vi "DO redefine.vi"(6 "conninfo":T3={"host"="localhost", "port"="5432", "client_encoding"="WIN1251", "dbname"="data", "user"="postgres", "password"=""}, 7 "KFM":string[](array[string]), 8 "error in (no error)":errorcluster, 9 "DOParamTable":string="fdo_3", 10 "DOParameters":string[](array[string]), 11 "DO in":T1) -> (0 "error":errorcluster, 3 "DO out":T1)   [LabVIEW 2019, in "Inputs.lvlib"]
uses:
  Inputs.lvlib
  Ctl/DO.ctl
  Ctl/Parameter State.ctl
  Database/ctl/Coninfo.ctl
  Ctl/DOParamColumns.ctl
  Database/select_initial.vi
  Database/PostgreSQL2LabVIEW/libpqUtility/src/PQclose.vi
  Database/PostgreSQL2LabVIEW/libpqUtility/src/PQconnect.vi
  Database/PostgreSQL2LabVIEW/libpqlv/src/PQfinish.vi
  Database/PostgreSQL2LabVIEW/libpqlv/src/PQconnectdb.vi
  Database/PostgreSQL2LabVIEW/libpqlv/src/PQerrorMessage.vi
  Database/PostgreSQL2LabVIEW/libpqlv/src/PQstatus.vi
  <vilib>/dlg_ctls.llb/Space Constant.vi
  Database/PostgreSQL2LabVIEW/libpqUtility/src/PQgetTable.vi
  Database/Progress.vi
  Database/PostgreSQL.lvlib
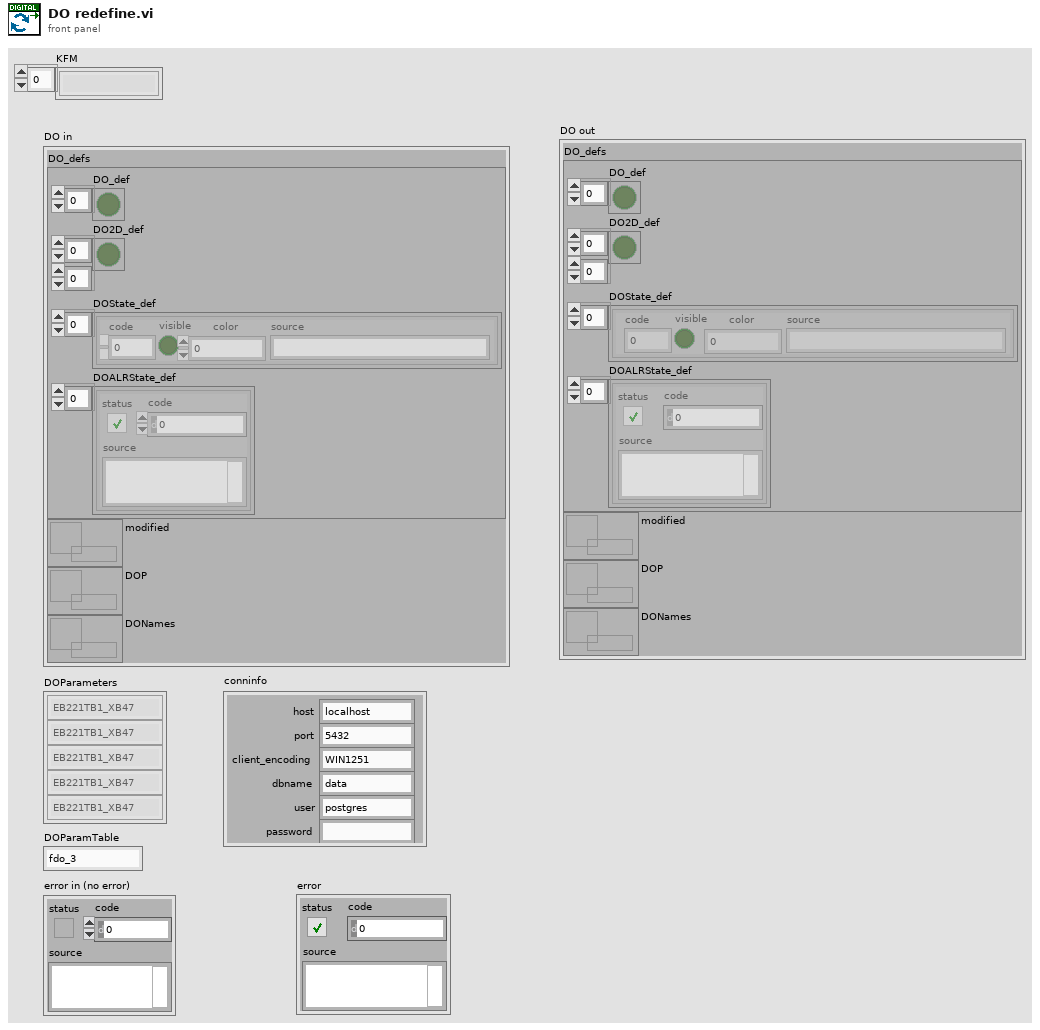
[diagram p1: front panel]
types:
  T1 = typedef "Inputs.lvlib/DO.ctl" = cluster{"DO_defs":cluster{"DO_def":bool[], "DO2D_def":bool[][], "DOState_def":T2[], "DOALRState_def":errorcluster[]}, "modified":refnum<data-value>, "DOP":refnum<data-value>, "DONames":refnum<data-value>}
  T2 = typedef "Inputs.lvlib/Parameter State.ctl" = cluster{"code":i32, "visible":bool, "color":u32, "source":string}
  T3 = typedef "PostgreSQL.lvlib/Coninfo.ctl" = cluster{"host":string, "port":string, "client_encoding":string, "dbname":string, "user":string, "password":string}
  T4 = typedef "Inputs.lvlib/DOParamColumns.ctl" = enum16{"module_fcode_full", "control_channel_num", "fcode", "fcodef", "fcode_full", "fname"}
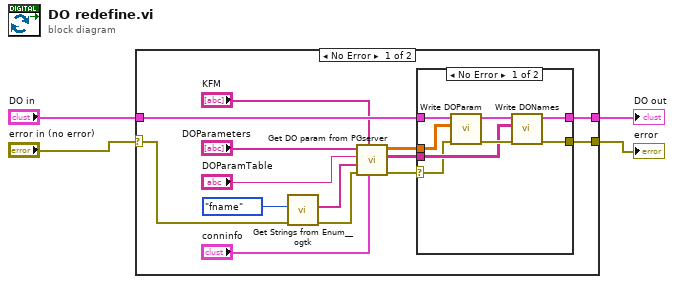
[diagram p0: block diagram]
diagram:
  n1 = case shown="No Error" "error in (no error)" {
    selector: "error in (no error)" -> [w7 w30]
    tunnel: [w13 w30] -> w4
    tunnel: "DO in" -> [w11 w29]
    tunnel: [w10 w29] -> w3
    frame No Error {
      n2 = call <userlib>:"Get Strings from Enum__ogtk.vi"("error in (no error)"=w7, "Enum"=DOParamColumns."fname" ("DOParamColumns")) -> ("error out"=w6:errorcluster, "Enum Strings"=w5:string[])  [unwired: 6 in, 2 out]
      n3 = call "Get DO param from PGserver.vi"("conninfo"="conninfo", "KFM"="KFM", "error in (no error)"=w6, "DOParamColumns"=w5, "DOParamTable"="DOParamTable", "DO_fcode_full"="DOParameters") -> ("error out"=w15:errorcluster, "Names table"=w16:string[][], "DOParameters table"=w17:dbl[][])  [unwired: 3 in]
      n4 = case shown="No Error" w15 {
        selector: w15 -> [w19 w27]
        tunnel: w17 -> [w20 _]
        tunnel: w16 -> [w21 _]
        tunnel: [w23 w27] -> w13
        tunnel: w11 -> [w26 w28]
        tunnel: [w22 w28] -> w10
        frame No Error {
          n5 = call "Write DOParam.vi"("error in (no error)"=w19, "DOParam"=w20, "DO in"=w26) -> ("error out"=w24:errorcluster, "DO out"=w25:T1)  [unwired: 7 in]
          n6 = call "Write DONames.vi"("error in (no error)"=w24, "DONames"=w21, "DO in"=w25) -> ("error out"=w23:errorcluster, "DO out"=w22:T1)  [unwired: 7 in]
        }
        frame Error {
        }
      }
    }
    frame Error {
    }
  }
  "DO out" <- w3
  "error" <- w4
